vi "Four Probe Asynchronous.vi"(10 "Error Stream gRPCid":T1, 11 "gRPCid":T1) -> ()   [LabVIEW 2019]
uses:
  VIs/MeasurementServer_gRPCid.ctl
  Global Operations.ctl
  VIs/labview-grpc-measurement-server.lvlib
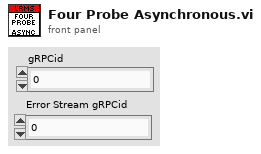
[diagram p1: front panel]
types:
  T1 = typedef "labview-grpc-measurement-server.lvlib/MeasurementServer_gRPCid.ctl" = u64
  T2 = typedef "Global Operations.ctl" = enum16{"Get", "Set"}
  T3 = typedef "labview-grpc-measurement-server.lvlib/MeasurementServer_FourProbeRawData.ctl" = cluster{"Positive Voltage":dbl, "Positive Current":dbl, "Negative Voltage":dbl, "Negative Current":dbl, "Impedance":dbl, "ErrorOutData":T4}
  T4 = typedef "labview-grpc-measurement-server.lvlib/MeasurementServer_ErrorOutData.ctl" = cluster{"ErrorCode":i32, "ErrorMessage":string}
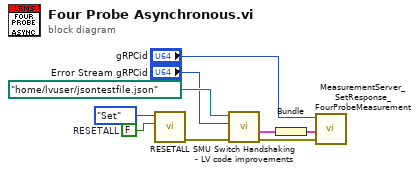
[diagram p0: block diagram]
diagram:
  w5 = FALSE  # RESETALL
  n1 = call "RESETALL.vi"("RESETALL"=w5, "Operation"=Global_Operations."Set") -> ("error out"=w3:errorcluster)  [unwired: 8 in, 1 out]
  n2 = call "SMU Switch Handshaking - LV code improvements.vi"("error in"=w3, "Error Stream gRPCid"="Error Stream gRPCid", "file path (use dialog)"=path "/home/lvuser/jsontestfile.json") -> ("error out"=w2:errorcluster, "Results"=w7:T3[])  [unwired: 6 in, 1 out]
  n3 = Bundle("Results"=w7) -> (w6:cluster{"Results":T3[]})  [unwired: 1 in]
  n4 = call "MeasurementServer_SetResponse_FourProbeMeasurement.vi"("gRPCid"="gRPCid", "FourProbeResponse"=w6, "error in (no error)"=w2) -> ()  [unwired: 7 in, 1 out]
